vi "Configure test.vi"(6 "Assert VI Path":path, 7 "Existing Queue Elements":string, 8 "error in (no error)":errorcluster, 11 "Floating Point in":refnum<class "Floating Point.lvclass">) -> (0 "error out":errorcluster, 3 "Floating Point out":refnum<class "Floating Point.lvclass">)   [LabVIEW 2018, in "Floating Point.lvclass"]
uses:
  Floating Point.lvclass
  <vilib>/Utility/Data Type/Type Definitions/Data Type.ctl
  Floating Point.lvclass/Floating Point.ctl
  5844b71f-7f9b-4df4-b9ee-b9122930f7bd.vi
  <vilib>/JDP Science/JSONtext/Find Item.vi
  5844b71f-7f9b-4df4-b9ee-b9122930f7bd.vi/7540fa09-2bb9-4f27-aca7-7263f7698e31.vi
  5844b71f-7f9b-4df4-b9ee-b9122930f7bd.vi/375e59cd-b435-4c76-a406-02a4f1021922.vi
  <vilib>/JDP Science/JSONtext/String Subset.vi
  Test Class String IDs.vi
  <vilib>/JDP Science/JSONtext/Parsing/Parse Full Path or Item Name.vi
  <vilib>/JDP Science/JSONtext/Offset/Find Item Locations by Path.vi
  <vilib>/JDP Science/JSONtext/JSON text to Variant.vi
  <vilib>/JDP Science/JSONtext/Variant to JSON Text.vi
  <vilib>/JDP Science/JSONtext/Set Item.vi
  Test.lvclass
  <vilib>/Utility/Data Type/NI_Data Type.lvlib
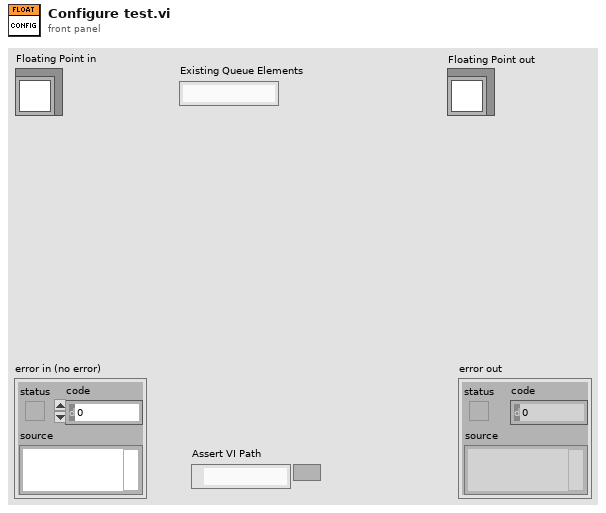
[diagram p1: front panel]
types:
  T1 = typedef "NI_Data Type.lvlib/Data Type.ctl" = enum8{"Invalid Type", "Void", "I8", "I16", "I32", "I64", "U8", "U16", "U32", "U64", "Single Float", "Double Float", "Extended Float", "Single Complex", "Double Complex", "Extended Complex", "Enum U8", "Enum U16", "Enum U32", "Enum U64", "Single Float With Unit", "Double Float With Unit", "Extended Float With Unit", "Single Complex with Unit", "Double Complex with Unit", "Extended Complex with Unit", "Boolean", "String", "Path", "Picture", "Tag", "Array", "Cluster", "Variant", "LV Variant", "Waveform", "Timestamp", "Digital Waveform", "Digital Data", "ExpressData", "Refnum", "External Data", "VI", "Poly VI", "LabVIEW Class Instance", "Fixed Point"}
  T2 = cluster{"Additional Data":string, "Comparison Value":string, "Invert?":string, "Assert Name":string, "Comment":string, "Default Failure Action":string, "Assert Build Timestamp":string, "Assert Builder User Name":string, "Data Type":string, "Assert VI Name":string, "Evaluation String":string}
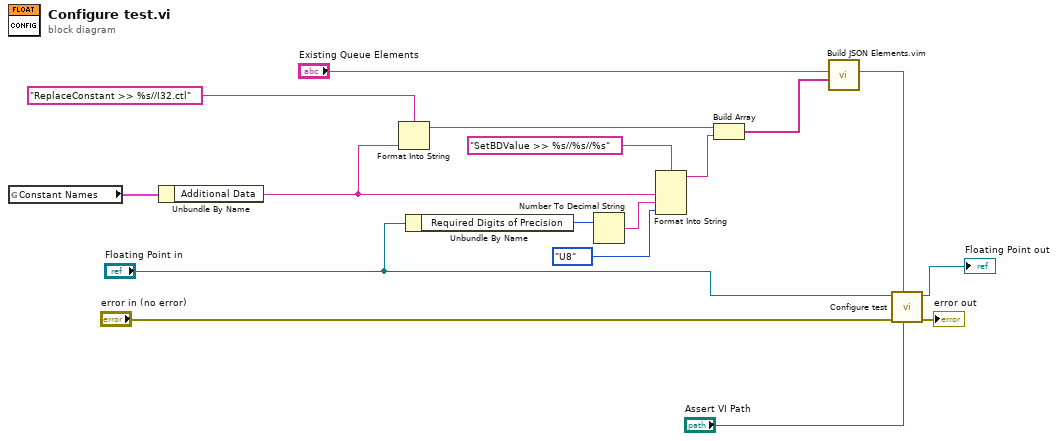
[diagram p0: block diagram]
diagram:
  n1 = global read "Test Class String IDs.vi" "Constant Names"() -> (w6:T2)
  n2 = Unbundle By Name(w6) -> ("Additional Data"=w2:string)
  n3 = Format Into String(format string="ReplaceConstant >> %s//I32.ctl" ("Append Element(s)"), w2) -> (resulting string=w7:string)  [unwired: 2 in, 1 out]
  n4 = Unbundle By Name("Floating Point in") -> ("Required Digits of Precision"=w5:u8)
  n5 = Number To Decimal String(number=w5) -> (decimal integer string=w4:string)  [unwired: 1 in]
  n6 = Format Into String(format string="SetBDValue >> %s//%s//%s", w2, w4, Data_Type."U8" ("input 3")) -> (resulting string=w12:string)  [unwired: 2 in, 1 out]
  n7 = Build Array(w7, w12) -> (w11:string[])
  n8 = call "Build JSON Elements.vim"("Append Element(s)"=w11, "JSON Elements in ({})"="Existing Queue Elements") -> ("JSON Elements out"=w9:string)  [unwired: 9 in]
  n9 = call-parent "Configure test.vi"("Assert VI Path"="Assert VI Path", "Existing Queue Elements"=w9, "error in (no error)"="error in (no error)", "Basic Test in"="Floating Point in") -> ("error out"=→"error out":errorcluster, "Test out"=→"Floating Point out":refnum<class "Floating Point.lvclass">)  [unwired: 6 in]
